vi "test Read I32 Array.vi"(8 "error in (no error)":errorcluster, 11 "TestCase in":refnum<class "Buffer Tests.lvclass">) -> (0 "error out":errorcluster, 3 "TestCase out":refnum<class "Buffer Tests.lvclass">)   [LabVIEW 2017, in "Buffer Tests.lvclass"]
uses:
  Buffer Tests.lvclass
  <vilib>/NI/Memory Manager/Classes/Pointer/Pointer.lvclass/Pointer.ctl
  <vilib>/NI/Memory Manager/Classes/Pointer/Get Internal.vi
  <vilib>/NI/Memory Manager/Classes/Pointer/Errors.vi
  <vilib>/NI/Memory Manager/Classes/Pointer/Zone.vi
  <vilib>/NI/Memory Manager/Classes/Pointer/Set Address.vi
  <vilib>/NI/Memory Manager/Classes/Pointer/Set Size.vi
  <vilib>/NI/Memory Manager/Classes/Pointer/Set Internal.vi
  <vilib>/NI/Memory Manager/Classes/Pointer/Get Address.vi
  <vilib>/NI/Memory Manager/Classes/Pointer/Check Null Pointer.vi
  <vilib>/NI/Memory Manager/Classes/Pointer/Create Error.vi
  <vilib>/NI/Memory Manager/Classes/Pointer/Null Pointer.vi
  <vilib>/NI/Memory Manager/Classes/Pointer/Is Null.vi
  <vilib>/NI/Memory Manager/Constants/Constants.vi
  <vilib>/NI/Memory Manager/Constants/Library Name.vi
  <vilib>/NI/Memory Manager/Classes/Pointer/Pointer Error Info.vi
  <vilib>/NI/Memory Manager/Constants/Pointer Class Name.vi
  Classes/Buffer/Buffer.lvclass
  C:/Program Files (x86)/National Instruments/LabVIEW 2017/vi.lib/NI/Memory Manager/Classes/Pointer/Pointer.lvclass
  Classes/Buffer/Read Buffer 1D I32.vi
  <vilib>/NI/Memory Manager/VIs/New Error Cluster.vi
  <vilib>/NI/Memory Manager/VIs/New Error Cluster (512B).vi
  <vilib>/NI/Memory Manager/VIs/Set Error Status.vi
  <vilib>/NI/Memory Manager/VIs/Set Error Code.vi
  <vilib>/NI/Memory Manager/VIs/Set Error Source.vi
  <vilib>/NI/Memory Manager/VIs/Write String to Source.vi
  <vilib>/addons/_JKI Toolkits/VI Tester/TestCase.llb/TestCase.lvclass
  <vilib>/NI/Memory Manager/Classes/Pointer/Pointer.lvclass
  C:/Program Files (x86)/National Instruments/LabVIEW 2017/vi.lib/addons/_JKI Toolkits/VI Tester/TestCase.llb/TestCase.lvclass
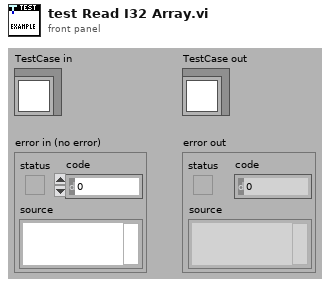
[diagram p1: front panel]
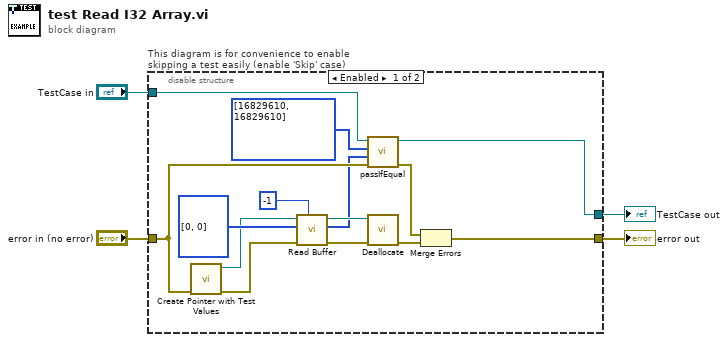
[diagram p0: block diagram]
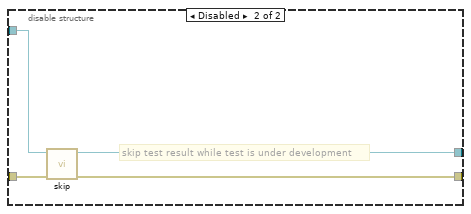
[diagram p2: hidden frame]
diagram:
  n1 = disable-structure "This diagram is for convenience to enable skipping a test easily (enable 'Skip' case)" shown="Enabled" {
    disable-tunnel: "TestCase in" -> [w14 w22]
    disable-tunnel: [w15 w20] -> w1
    disable-tunnel: [w12 w21] -> w2
    disable-tunnel: "error in (no error)" -> [w13 w19]
    frame Enabled {
      n2 = call "Create Pointer with Test Values.vi"("error in (no error)"=w13) -> ("error out"=w7:errorcluster, "Buffer out"=w6:refnum<class "Buffer.lvclass">)  [unwired: 9 in]
      n3 = call-poly "Read Buffer.vi"("count (-1: rest)"=i64 -1 ("count"), "error in (no error)"=w7, "dst array in"=i32[] [0, 0] ("buffer in"), "Buffer in"=w6) -> ("error out"=w17:errorcluster, "dst array out"=w9:i32[], "Buffer out"=w18:refnum<class "Buffer.lvclass">)  [unwired: 4 in, 1 out]
      n4 = call-dynamic "passIfEqual.vi"("error in (no error)"=w13, "y"=w9, "x"=i32[] [16829610, 16829610] ("reversed array 2"), "TestCase in"=w14) -> ("error out"=w16:errorcluster, "TestCase out"=w15:refnum<class "Buffer Tests.lvclass">)  [unwired: 6 in]
      n5 = call <vilib>:"Deallocate.vi"("error in (no error)"=w17, "Pointer"=w18) -> ("error out"=w5:errorcluster)  [unwired: 8 in, 1 out]
      n6 = Merge Errors(w16, w5) -> (w12:errorcluster)
    }
    frame Disabled {
      # "skip test result while test is under development"
      n7 = call <vilib>:"skip.vi"("error in (no error)"=w19, "TestCase in"=w22) -> ("error out"=w21:errorcluster, "TestCase out"=w20:refnum<class "Buffer Tests.lvclass">)  [unwired: 8 in]
    }
  }
  "error out" <- w2
  "TestCase out" <- w1
